vi "ProdaNG.Configurator.Glb.vi"() -> ()   [LabVIEW 2016]
uses:
  Controls/ProdaNG.TestStep.ctl
  Controls/ProdaNG.TestStepParam.ctl
  Controls/ProdaNG.TestValue.ctl
  Controls/ProdaNG.ProcessStepParam.ctl
  Controls/ProdaNG.System.ctl
  Controls/ProdaNG.WabcoPart.ctl
  Controls/ProdaNG.ProdutionLine.ctl
  Controls/ProdaNG.Process.ctl
  ProdaNG.Configurator.Config.ctl
panel:
  in  "Configuration":T1={"ShowUnreleased"=TRUE, "Param1"="StepIndex", "ParamStartIdx"=0, "Slots"=1} {"Slots" min=1 max=2; "ParamStartIdx" min=0 max=1}
  in  "Processes":T2[](array[typedef])
  out "ProdLines":T3[](array[typedef])
  in  "WabcoParts":T4[](array[typedef])
  in  "Systems":T5[](array[typedef])
  out "TSrelease":T6[](array[typedef])
  out "PP":T7[](array[typedef])
  out "TS":cluster{"TS":T6, "TP":T8[], "TV":T9[]}[](array[cluster]) {"TV"."minimum" format="%#.3f"; "TV"."maximum" format="%#.3f"; "TP"."value" format="%#.3f"}
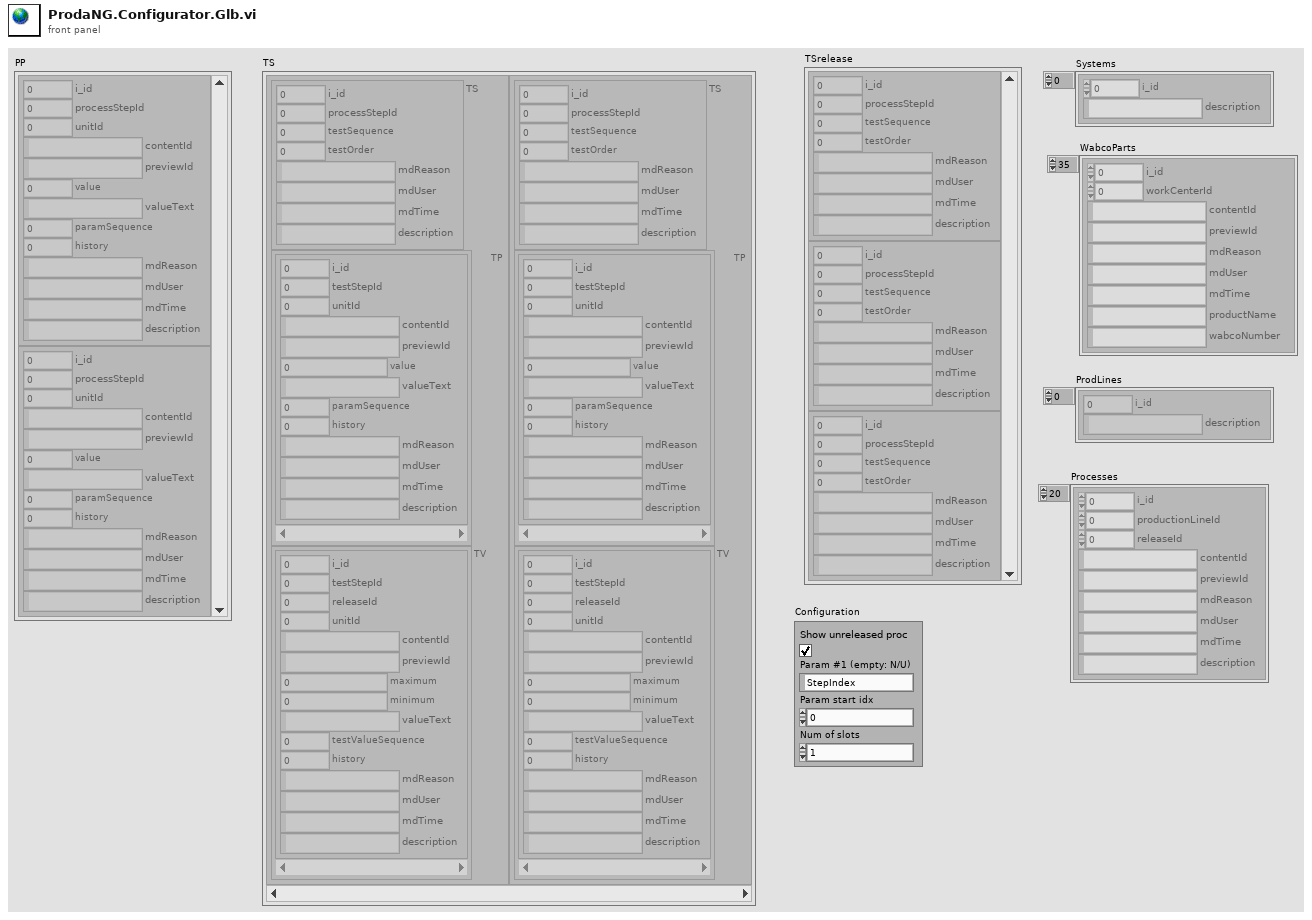
[diagram p1: front panel]
types:
  T1 = typedef "ProdaNG.Configurator.Config.ctl" = cluster{"ShowUnreleased":bool, "Param1":string, "ParamStartIdx":i32, "Slots":i32}
  T2 = typedef "ProdaNG.Process.ctl" = cluster{"i_id":i32, "productionLineId":i32, "releaseId":i32, "contentId":string, "previewId":string, "mdReason":string, "mdUser":string, "mdTime":string, "description":string}
  T3 = typedef "ProdaNG.ProdutionLine.ctl" = cluster{"i_id":i32, "description":string}
  T4 = typedef "ProdaNG.WabcoPart.ctl" = cluster{"i_id":i32, "workCenterId":i32, "contentId":string, "previewId":string, "mdReason":string, "mdUser":string, "mdTime":string, "productName":string, "wabcoNumber":string}
  T5 = typedef "ProdaNG.System.ctl" = cluster{"i_id":i32, "description":string}
  T6 = typedef "ProdaNG.TestStep.ctl" = cluster{"i_id":i32, "processStepId":i32, "testSequence":i32, "testOrder":i32, "mdReason":string, "mdUser":string, "mdTime":string, "description":string}
  T7 = typedef "ProdaNG.ProcessStepParam.ctl" = cluster{"i_id":i32, "processStepId":i32, "unitId":i32, "contentId":string, "previewId":string, "value":dbl, "valueText":string, "paramSequence":i32, "history":i32, "mdReason":string, "mdUser":string, "mdTime":string, "description":string}
  T8 = typedef "ProdaNG.TestStepParam.ctl" = cluster{"i_id":i32, "testStepId":i32, "unitId":i32, "contentId":string, "previewId":string, "value":dbl, "valueText":string, "paramSequence":i32, "history":i32, "mdReason":string, "mdUser":string, "mdTime":string, "description":string}
  T9 = typedef "ProdaNG.TestValue.ctl" = cluster{"i_id":i32, "testStepId":i32, "releaseId":i32, "unitId":i32, "contentId":string, "previewId":string, "maximum":dbl, "minimum":dbl, "valueText":string, "testValueSequence":i32, "history":i32, "mdReason":string, "mdUser":string, "mdTime":string, "description":string}
diagram:
